vi "MAT_Get_HB0_filter_coefficients.vi"(1 "1st order derivative? (F)":bool, 2 "N":i32=5 min=5 max=31 step=2) -> (0 "HB smoothing filter coefficients (exact up to x^4)":dbl[](array[numeric])=[-0.0625, 0.25, 0.625, 0.25, -0.0625])   [LabVIEW 2018, in "Tracker.lvlib"]
uses:
  Tracker.lvlib
  <vilib>/gmath/NI_Gmath.lvlib
panel:
  in  "Mult (check only)":dbl=1.0 format="%#_13g"
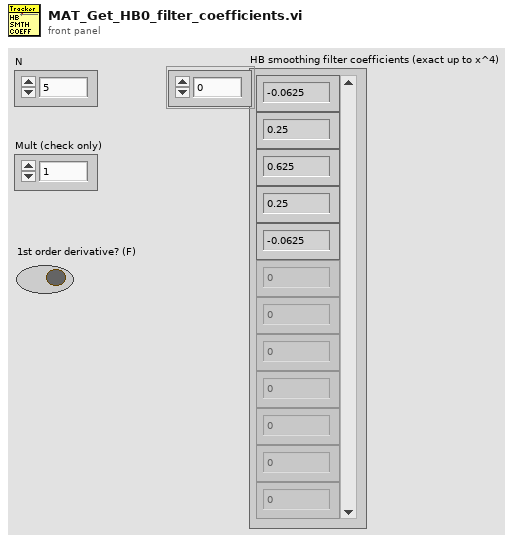
[diagram p1: front panel]
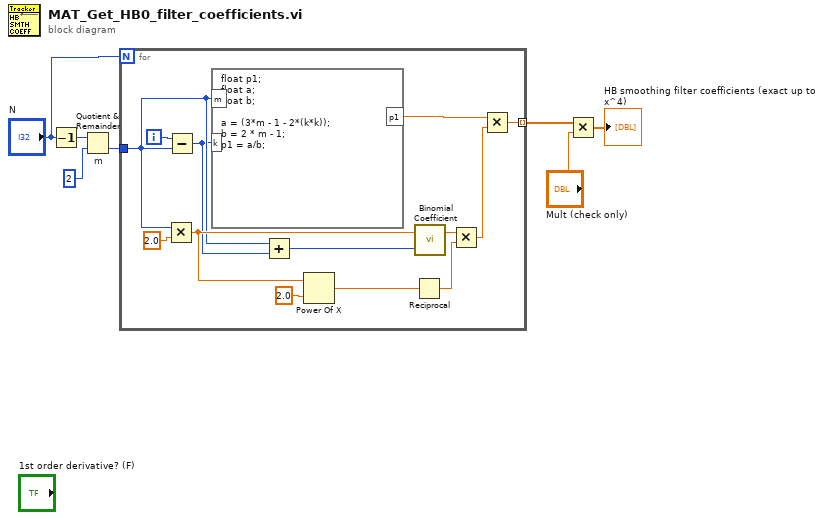
[diagram p0: block diagram]
diagram:
  n1 = Decrement(x="N") -> (x-1=w7:i32)
  n2 = Quotient & Remainder "m"(x=w7, y=2) -> (floor(x/y)=w5:i32)  [unwired: 1 out]
  n3 = for {
    N: "N" -> [_]
    tunnel: w5 -> [w9]
    tunnel: [w11] -> w3 mode=indexing
    i -> [w10]
    n4 = Multiply(x=w9, y=2.0 ("x")) -> (x*y=w12:dbl)
    n5 = Subtract(x=w10, y=w9) -> (x-y=w8:i32)
    n6 = formula code="float p1;\nfloat a;\nfloat b;\n\na = (3*m - 1 - 2*(k*k));\nb = 2 * m - 1;\np1 = a/b;"("m"=w9, "k"=w8) -> ("p1"=w15:dbl)
    n7 = Add(x=w9, y=w8) -> (x+y=w17:i32)
    n8 = Power Of X(1:2.0 ("y"), 2:w12) -> (0:w19:dbl)
    n9 = Reciprocal(x=w19) -> (1/x=w18:dbl)
    n10 = call <vilib>:"Binomial Coefficient.vi"("k"=w17, "n"=w12) -> ("binomial coefficient (n,k)"=w16:dbl)  [unwired: 1 out]
    n11 = Multiply(x=w16, y=w18) -> (x*y=w14:dbl)
    n12 = Multiply(x=w15, y=w14) -> (x*y=w11:dbl)
  }
  n13 = Multiply(x=w3, y="Mult (check only)") -> (x*y=→"HB smoothing filter coefficients (exact up to x^4)":dbl[])
